vi "Leja Order Roots (DBL).vi"(11 "Roots":dbl[](array[numeric])) -> (3 "Roots of Leja Order":dbl[](array[numeric]))   [LabVIEW 2018, in "NI_AALPro.lvlib"]
uses:
  <vilib>/Analysis/NI_AALPro.lvlib
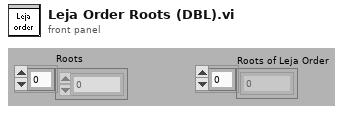
[diagram p1: front panel]
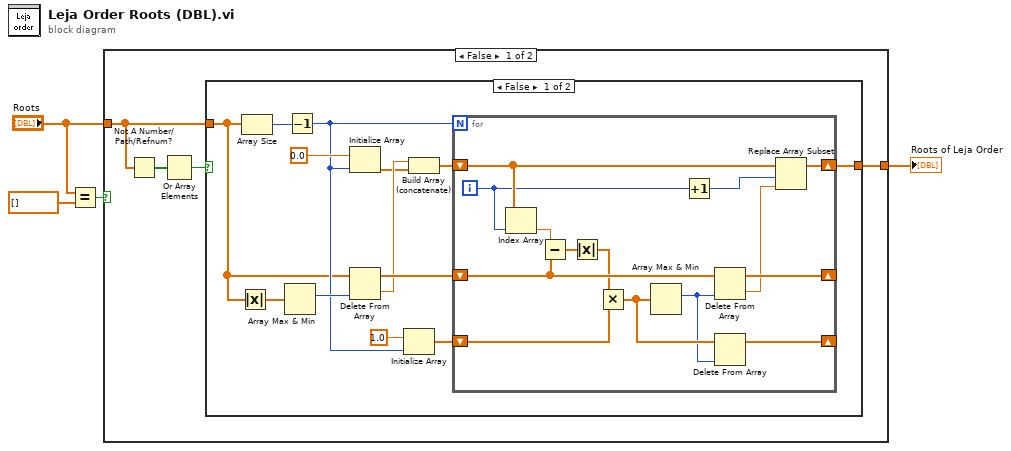
[diagram p0: block diagram]
diagram:
  n1 = Equal?(x="Roots", y=dbl[] []) -> (x = y?=w1:bool)
  n2 = case shown="False" w1 {
    tunnel: [w8 _] -> w4
    tunnel: "Roots" -> [w7 _]
    frame False {
      n3 = Not A Number/Path/Refnum?(number/path/refnum=w7) -> (NaN/Path/Refnum?=w6:bool[])
      n4 = Or Array Elements(Boolean array=w6) -> (logical OR=w5:bool)
      n5 = case shown="False" w5 {
        tunnel: [w16 w36] -> w8
        tunnel: w7 -> [w9 w36]
        frame False {
          n6 = Absolute Value(x=w9) -> (abs(x)=w21:dbl[])
          n7 = Array Size(array=w9) -> (size(s)=w18:i32)
          n8 = Array Max & Min(array=w21) -> (max index (indices)=w20:i32)  [unwired: 3 out]
          n9 = Decrement(x=w18) -> (x-1=w12:i32)
          n10 = Initialize Array(0.0 ("element"), w12) -> (w13:dbl[])
          n11 = Delete From Array(array=w9, index=w20) -> (deleted portion=w15:dbl, array with subset deleted=w19:dbl[])  [unwired: 1 in]
          n12 = Initialize Array(1.0, w12) -> (w10:dbl[])
          n13 = Build Array (concatenate)(w15, w13) -> (w17:dbl[])
          n14 = for {
            N: w12 -> [_]
            shift-right: [w34] -> w16
            shift-left: w17 -> [w31]
            shift-right: [w35] -> _
            shift-left: w19 -> [w29]
            shift-right: [w25] -> _
            shift-left: w10 -> [w22]
            i -> [w30]
            n15 = Index Array(array=w31, index=w30) -> (element=w28:dbl)
            n16 = Subtract(x=w28, y=w29) -> (x-y=w27:dbl[])
            n17 = Absolute Value(x=w27) -> (abs(x)=w23:dbl[])
            n18 = Multiply(x=w23, y=w22) -> (x*y=w26:dbl[])
            n19 = Array Max & Min(array=w26) -> (max index (indices)=w24:i32)  [unwired: 3 out]
            n20 = Increment(x=w30) -> (x+1=w32:i32)
            n21 = Delete From Array(array=w29, index=w24) -> (deleted portion=w33:dbl, array with subset deleted=w35:dbl[])  [unwired: 1 in]
            n22 = Delete From Array(array=w26, index=w24) -> (array with subset deleted=w25:dbl[])  [unwired: 1 in, 1 out]
            n23 = Replace Array Subset(array=w31, new element=w33, index=w32) -> (w34:dbl[])
          }
        }
        frame True {
        }
      }
    }
    frame True {
    }
  }
  "Roots of Leja Order" <- w4
